vi "Plot Editor.vi"(6 "Original Plot Idx":i32=-1, 7 "Original Graph Name":string, 8 "Error In":errorcluster, 9 "Plot Style in":T2={"Plot Index"=0, "Plot.Bar Plot Style"=0, "Plot.DigitalLineStyle"=1, "Plot.TransitionLocation"=2, "Plot.Transition Type"=0, "Plot.Fill To"=-1, "Plot.Fill/Pt. Color"=16777222, "Plot.Label Format"=3, "Plot.Line Style"=0, "Plot.Line Width"=1, "Plot.Plot Color"=16777222, "Plot.Plot Interpolation"=2, "Plot.Plot Name"="", "Plot.Point Style"=0, "Plot.Visible?"=TRUE, "Plot.XScaleIdx"=0, "Plot.YScaleIdx"=0, "Plot.Anti-aliased"=TRUE}, 10 "Plot in":T3, 11 "Original Graph Refnum":T1) -> (0 "Error Out":errorcluster, 1 "Plot Style out":T2, 2 "Plot out":T3)   [LabVIEW 2019, in "Plot Editor.lvlib"]
uses:
  Plot Editor.lvlib
  XY Graph/XY Graph Plot Properties.ctl
  XY Graph/XY Plot Data.ctl
  XY Graph/XY Graph Refnum.ctl
  Plot Editor Q [Element].ctl
  Plot Editor Q [Event] List.ctl
  Plot Editor Internal Variables.ctl
  <vilib>/Utility/error.llb/DialogType.ctl
  <vilib>/Utility/miscctls.llb/LVPoint32TypeDef.ctl
  XY Graph/XY Graph Add-Ons.lvlib
  Notebook/Notebook.lvlib
  Arrays/Define Ramp Array Dialog.vi
  Rich Text Box/Rich Text Box.lvlib
  Variant/Variant to Data/Variant to Data.lvlib
panel:
  out "Y Array Sum":dbl format="%#_5g"
  out "X Array Sum":dbl format="%#_5g"
  in  "X Array":dbl[](array[numeric])
  in  "Copy":bool
  in  "Cancel":bool
  out "Error":errorcluster
  in  "Reset Style":bool
  out "Y Array Size":i32 format="%#_5g"
  in  "Cancel Data Edit":bool
  in  "OK":bool
  out "X Array Size":i32 format="%#_5g"
  in  "Y Array":dbl[](array[numeric]) caption="X Array"
  out "Plot Preview":cluster{"X Array":dbl[], "Y Array":dbl[]}[](graph)
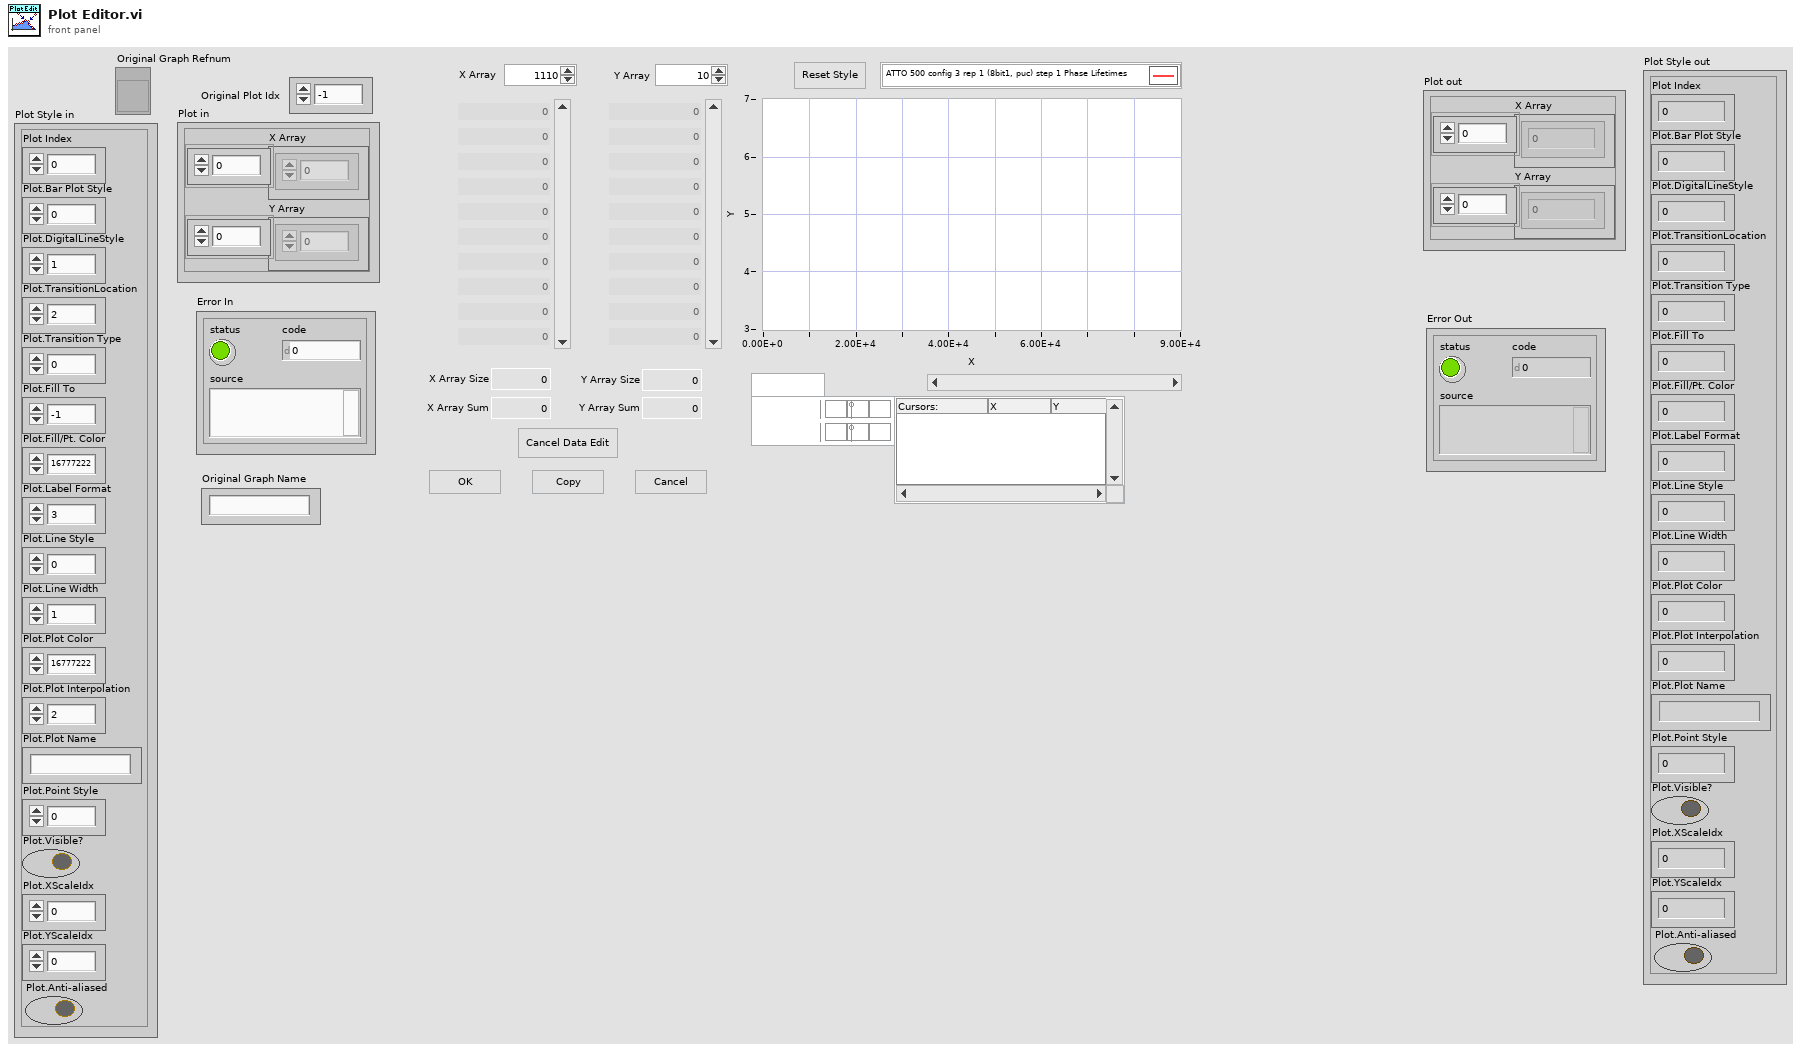
[diagram p1: front panel]
types:
  T1 = typedef "XY Graph Add-Ons.lvlib/XY Graph Refnum.ctl" = refnum<vi>
  T2 = typedef "XY Graph Plot Properties.ctl" = cluster{"Plot Index":i32, "Plot.Bar Plot Style":u8, "Plot.DigitalLineStyle":u8, "Plot.TransitionLocation":u8, "Plot.Transition Type":u8, "Plot.Fill To":i16, "Plot.Fill/Pt. Color":u32, "Plot.Label Format":u8, "Plot.Line Style":u8, "Plot.Line Width":u8, "Plot.Plot Color":u32, "Plot.Plot Interpolation":u8, "Plot.Plot Name":string, "Plot.Point Style":u8, "Plot.Visible?":bool, "Plot.XScaleIdx":u32, "Plot.YScaleIdx":u32, "Plot.Anti-aliased":bool}
  T3 = typedef "XY Plot Data.ctl" = cluster{"X Array":dbl[], "Y Array":dbl[]}
  T4 = typedef "Plot Editor.lvlib/Plot Editor Q [Element].ctl" = cluster{"Plot Editor Q Event":T5, "Data":variant}
  T5 = typedef "Plot Editor.lvlib/Plot Editor Q [Event] List.ctl" = enum16{"Idle", "Initialization", "Controls >> Store", "Store >> Plot", "Update Plot Style", "Check Data Array Alignment", "Reset Data", "Reset Style", "Accept & Quit", "Copy & Quit", "Save Plot", "Load Plot", "Remove out-of-bound Values", "Delete Element", "Insert Element Before", "Insert Element After", "Update output string", "Remove NaN-containing Pairs", "Fill Array with Ramp", "Quit"}
  T6 = typedef "Plot Editor.lvlib/Plot Editor Internal Variables.ctl" = cluster{"X Array":dbl[], "Y Array":dbl[], "XY Plot Properties":T2, "X Array Index Values":u32[], "Y Array Index Values":u32[], "Original XY Plot Properties":T2, "Original X Array":dbl[], "Original Y Array":dbl[], "VI title suffix":string, "Refnum based call":bool}
  T7 = typedef "LVPoint32TypeDef.ctl" = cluster{"Horizontal":i32, "Vertical":i32}
  T8 = typedef "Rich Text Box.lvlib/Text Formatting.ctl" = cluster{"Font":string, "Text Color":T9, "Text Background Color":T9, "Text Style":enum16{"Regular", "Bold", "Italic", "Underline", "Strikeout"}, "Font Size (Points)":dbl, "Text Alignment":i32}
  T9 = typedef "Rich Text Box.lvlib/Text Colors.ctl" = enum16{"Unchanged", "Black", "Blue", "Brown", "Gray", "Green", "Orange", "Pink", "Red", "White"}
  T10 = typedef "DialogType.ctl" = u16
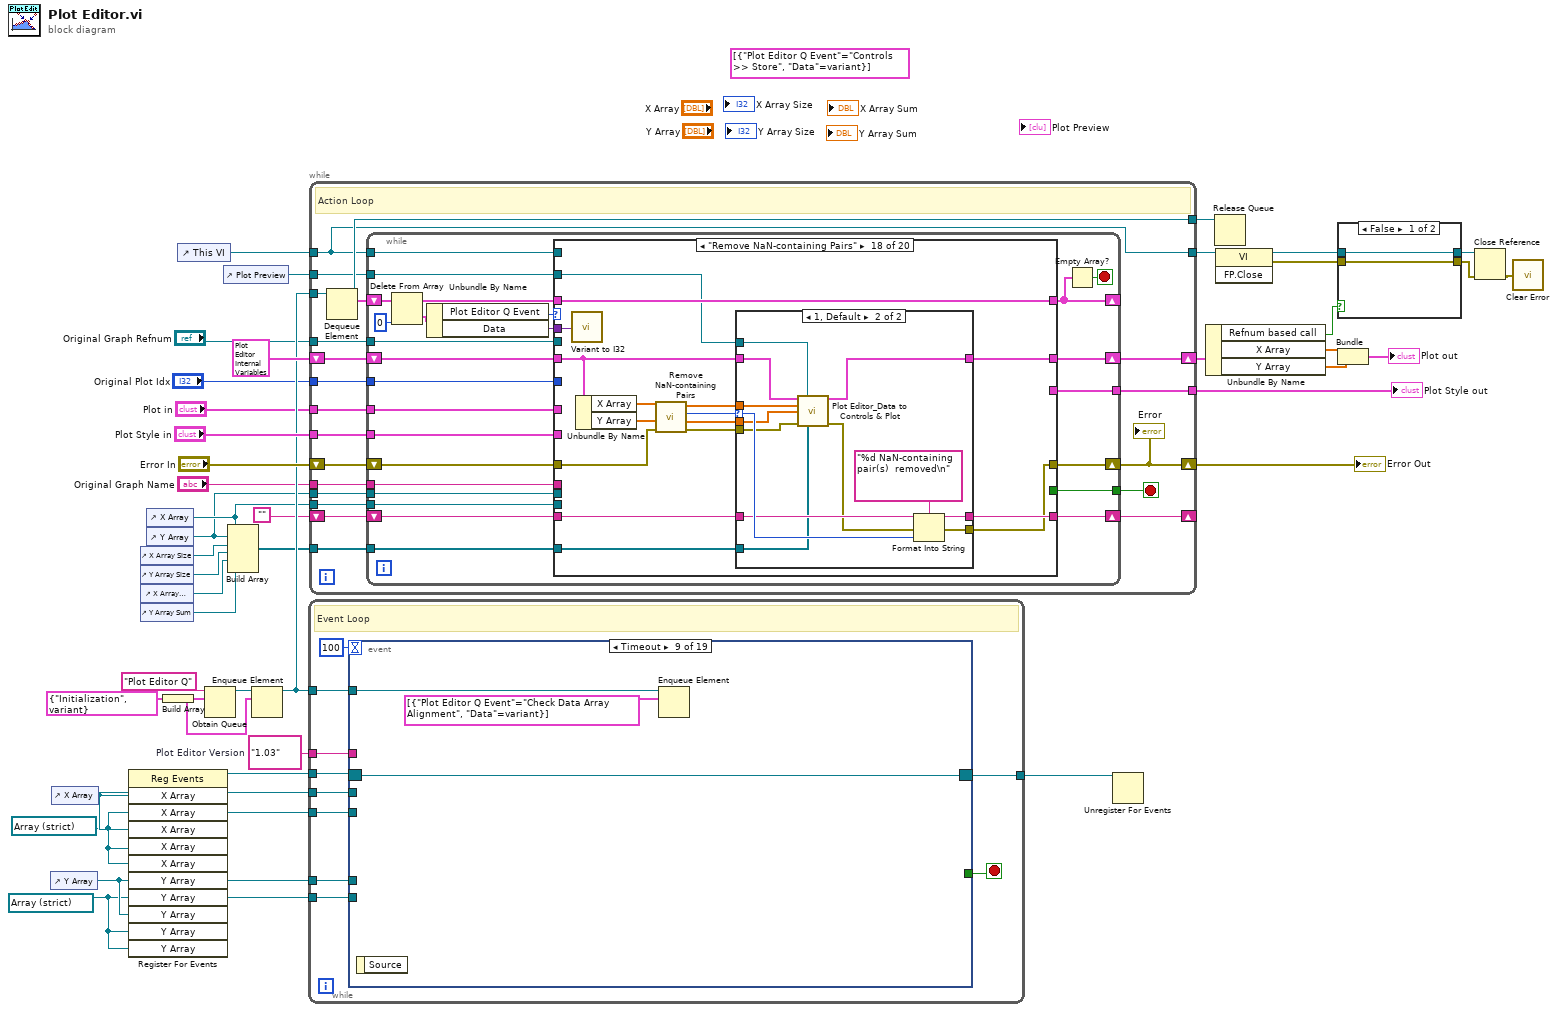
[diagram p0: block diagram]
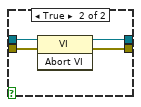
[diagram p2: hidden frame]
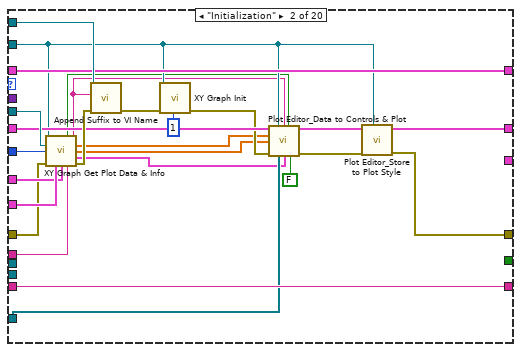
[diagram p4: hidden frame]
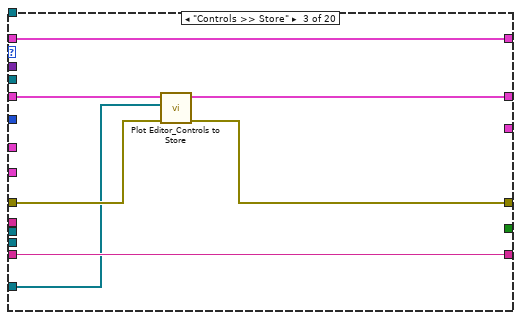
[diagram p5: hidden frame]
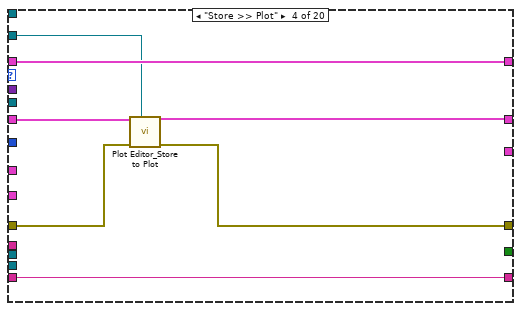
[diagram p6: hidden frame]
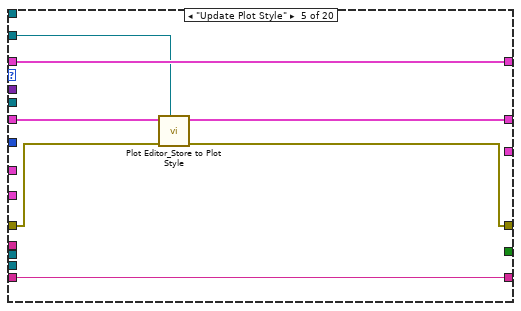
[diagram p7: hidden frame]
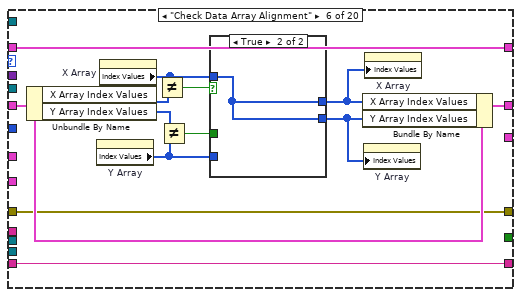
[diagram p8: hidden frame]
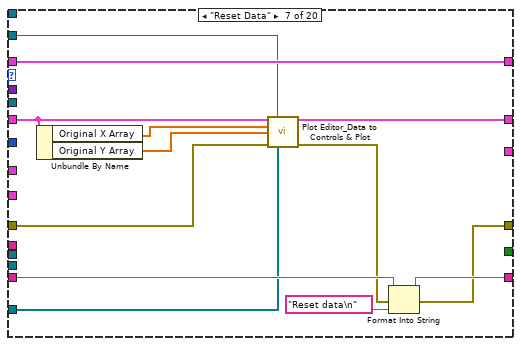
[diagram p11: hidden frame]
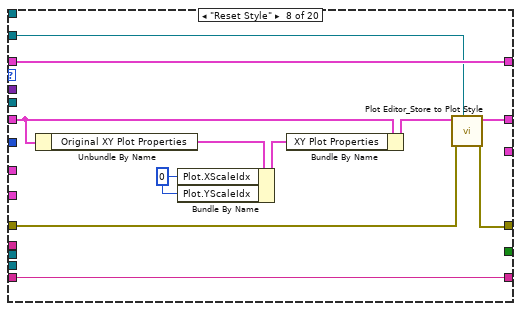
[diagram p12: hidden frame]
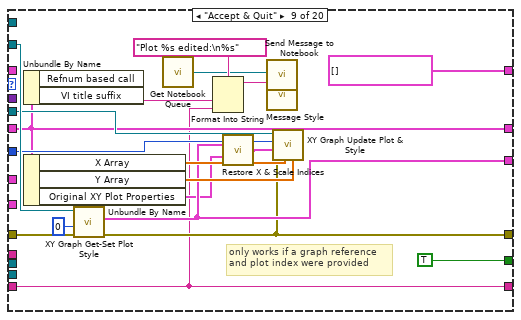
[diagram p13: hidden frame]
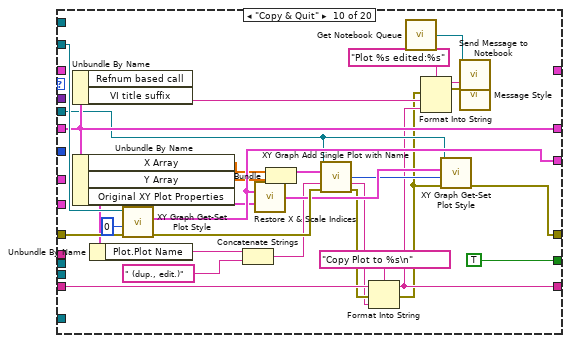
[diagram p14: hidden frame]
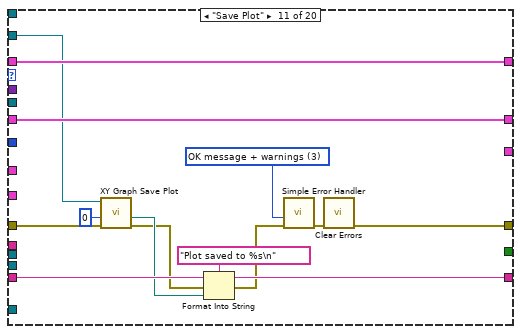
[diagram p15: hidden frame]
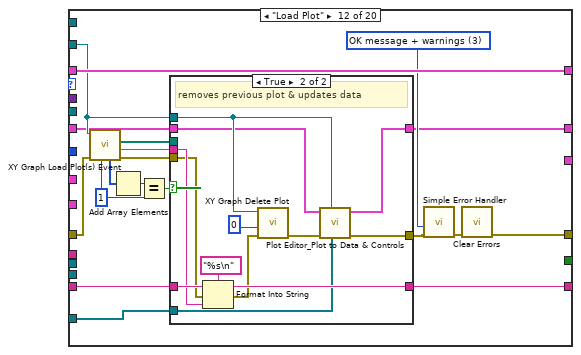
[diagram p16: hidden frame]
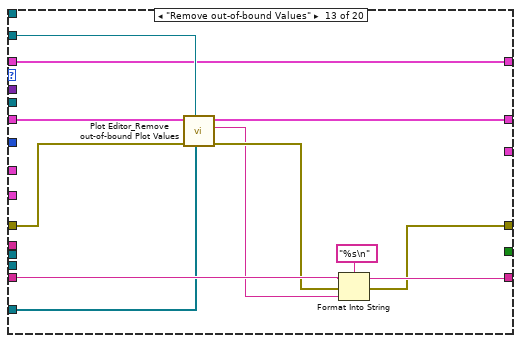
[diagram p18: hidden frame]
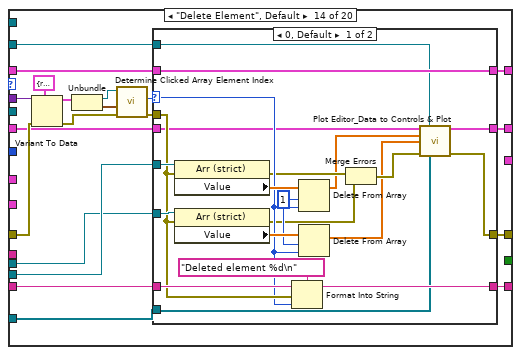
[diagram p19: hidden frame]
diagram:
  w4 = refnum<vi> refnum ("Y Array")
  w3 = refnum<vi> refnum ("X Array")
  (unwired) T4[] [{"Plot Editor Q Event"=enum."Controls >> Store", "Data"=variant}] ("array")
  w27 = "1.03"  # Plot Editor Version
  n1 = control-ref of="Y Array"() -> (w5:refnum<vi>)
  n2 = control-ref of="X Array"() -> (w6:refnum<vi>)
  n3 = register-events(w6, w3, w6, w3, w3, w5, w4, w5, w4, w4) -> (reference out=w26:refnum<event-registration>)  [unwired: 2 in, 1 out]
  n4 = control-ref of="X Array Size"() -> (w9:refnum<vi>)
  n5 = control-ref of="Y Array Size"() -> (w8:refnum<vi>)
  n6 = control-ref of="X Array Sum"() -> (w2:refnum<vi>)
  n7 = control-ref of="Y Array Sum"() -> (w1:refnum<vi>)
  n8 = control-ref of="X Array"() -> (w11:refnum<vi>)
  n9 = control-ref of="Y Array"() -> (w10:refnum<vi>)
  n10 = Build Array(T4 {"Plot Editor Q Event"=enum."Initialization", "Data"=variant} ("Plot Editor Q Element")) -> (w28:T4[])
  n11 = control-ref of="This VI"() -> (w18:refnum<vi>)
  n12 = Obtain Queue(name (unnamed)="Plot Editor Q", element data type=w28) -> (queue out=w41:refnum<queue>)  [unwired: 3 in, 2 out]
  n13 = control-ref of="Plot Preview"() -> (w36:refnum<vi>)
  n14 = Build Array(w11, w10, w9, w8, w2, w1) -> (w7:refnum<vi>[])
  n15 = Enqueue Element(queue=w41, element=w28) -> (queue out=w29:refnum<queue>)  [unwired: 2 in, 2 out]
  n16 = while {
    tunnel: w29 -> [w52]
    tunnel: w27 -> [w51]
    tunnel: w26 -> [w50]
    tunnel: w6 -> [w49]
    tunnel: w5 -> [w48]
    tunnel: [w47] -> w25
    tunnel: w3 -> [w46]
    tunnel: w4 -> [w45]
    stop <- w53 stop-if-true
    # "Event Loop"
    n17 = event shown="[8] Timeout" {
      selector: w50 -> [_ _ _ _ _ w159 w163 w166 w169 w175 w181 w185 w190 _ _ _ _ _ _]
      dyn-events: [_ _ _ _ _ w158 w162 w166 w169 w174 w180 w184 w189 _ _ _ _ _ _] -> w47
      timeout: 100 -> [_ _ _ _ _ _ _ _ _ _ _ _ _ _ _ _ _ _ _]
      tunnel: [w56 w58 _ _ _ _ _ _ _ _ _ _ _ _ _ _ TRUE ("Discard?") TRUE ("Discard?") TRUE ("Discard?")] -> w53
      tunnel: w52 -> [w55 w59 w93 w124 w148 _ _ w165 w168 w171 w176 _ _ w200 w202 w204 w207 w210 w213]
      tunnel: w51 -> [_ w57 _ _ _ _ _ _ _ _ _ _ _ _ _ _ _ _ _]
      tunnel: w49 -> [_ _ _ _ _ w157 _ _ _ w173 _ w183 w188 _ _ _ _ _ _]
      tunnel: w48 -> [_ _ _ _ _ _ w161 _ _ _ w178 _ w187 _ _ _ _ _ _]
      tunnel: w46 -> [_ _ _ _ _ w156 _ _ _ w172 _ w182 _ _ _ _ _ _ _]
      tunnel: w45 -> [_ _ _ _ _ _ w160 _ _ _ w179 _ w186 _ _ _ _ _ _]
      event Panel Close? {
        w56 = TRUE ("Discard?")
        n18 = event-data() -> ()  [unwired: 1 in, 1 out]
        n19 = Enqueue Element(queue=w55, element=T4[] [{"Plot Editor Q Event"=enum."Quit", "Data"=variant}]) -> ()  [unwired: 2 in, 3 out]
        n20 = event-data("Discard?"=w56) -> ()  [unwired: 1 in, 1 out]
      }
      event Menu Selection (User) {
        n21 = event-data() -> ("ItemTag"=w60:string)  [unwired: 1 in]
        n22 = case shown="\"About...\"" w60 {
          tunnel: w59 -> [_ w62 w64 w68 w81 _]
          tunnel: [_ _ _ w65 _ _] -> w58
          tunnel: w57 -> [_ _ _ _ _ w86]
          frame "", Default {
          }
          frame "Save Plot" {
            n23 = Enqueue Element(queue=w62, element=T4[] [{"Plot Editor Q Event"=enum."Save Plot", "Data"=variant}]) -> ()  [unwired: 2 in, 3 out]
          }
          frame "Load Plot" {
            n24 = Enqueue Element(queue=w64, element=T4[] [{"Plot Editor Q Event"=enum."Load Plot", "Data"=variant}]) -> ()  [unwired: 2 in, 3 out]
          }
          frame "Quit" {
            n25 = call "Two Buttons Dialog Window.vi"("OK Button Text"="Accept & Quit" ("T button name (\"OK\")"), "Message"="Are you sure you want to quit Plot Editor?\nQuitting will save the current changes and return to the original graph." ("message")) -> ("OK?"=w65:bool)  [unwired: 1 in]
            n26 = case shown="True" w65 {
              tunnel: w68 -> [_ w70]
              frame False {
              }
              frame True {
                n27 = Enqueue Element(queue=w70, element=T4[] [{"Plot Editor Q Event"=enum."Accept & Quit", "Data"=variant}]) -> ()  [unwired: 2 in, 3 out]
              }
            }
          }
          frame "Paste Data from Clipboard" {
            w72 = "\n"
            n28 = invoke class="App" method="Clipboard.Read"() -> ("Read Clipbrd"=w78:string)  [unwired: 3 in, 2 out]
            n29 = call <userlib>:"String to 1D Array__ogtk.vi"("delimiter (Tab)"=w72, "string"=w78) -> ("Array of Strings"=w77:string[])  [unwired: 9 in]
            n30 = Delete From Array(array=w77, length=1, index=0) -> (array with subset deleted=w74:string[])  [unwired: 1 out]
            n31 = call <userlib>:"1D Array to String__ogtk.vi"("delimiter (Tab)"=w72, "Array of Strings"=w74) -> ("delimited string"=w73:string)  [unwired: 9 in]
            n32 = Spreadsheet String To Array(format string="%#g", spreadsheet string=w73) -> (array=w84:dbl[][])  [unwired: 2 in]
            n33 = Transpose 2D Array(2D array=w84) -> (transposed array=w71:dbl[][])
            n34 = Enqueue Element(queue=w81, element=T4[] [{"Plot Editor Q Event"=enum."Controls >> Store", "Data"=variant}, {"Plot Editor Q Event"=enum."Store >> Plot", "Data"=variant}]) -> ()  [unwired: 2 in, 3 out]
            n35 = Index Array(array=w71) -> (element #1=w83:dbl[], element #2=w82:dbl[])  [unwired: 4 in]
            n36 = local write "X Array"(w83) -> ()
            n37 = local write "Y Array"(w82) -> ()
          }
          frame "About..." {
            n38 = Format Into String(format string="                                      Plot Editor\n                                      version %s\n\n                              Author: X. Michalet\n(c) 2017-2020 The Regents of the  University of California" ("message"), w86) -> (resulting string=w85:string)  [unwired: 2 in, 1 out]
            n39 = One Button Dialog(message=w85) -> ()  [unwired: 1 in, 1 out]
          }
        }
      }
      event "X Array": Shortcut Menu Selection (User) {
        n40 = event-data() -> ("ItemTag"=w94:string, "CtlRef"=w91:refnum<vi>, "Coords"=w90:T7)  [unwired: 1 in]
        n41 = case shown="\"Remove NaN-containing Pairs\"" w94 {
          tunnel: [w95 w101 w107 w113 w116 w118] -> w92
          tunnel: w91 -> [_ w100 w106 w112 _ _]
          tunnel: w90 -> [_ w99 w105 w111 _ _]
          frame "", Default {
            n42 = Build Array(T4 {"Plot Editor Q Event"=enum."Idle", "Data"=variant} ("Plot Editor Q Element")) -> (w95:T4[])
          }
          frame "Delete Element" {
            n43 = Bundle("CtlRef"=w100, "Coords"=w99) -> (w97:cluster{"CtlRef":refnum<vi>, "Coords":T7})  [unwired: 1 in]
            n44 = Bundle By Name(cluster=T4 {"Plot Editor Q Event"=enum."Delete Element", "Data"=variant} ("Plot Editor Q Element"), "Data"=w97) -> (w98:T4)
            n45 = Build Array(w98) -> (w101:T4[])
          }
          frame "Insert Element Before" {
            n46 = Bundle("CtlRef"=w106, "Coords"=w105) -> (w103:cluster{"CtlRef":refnum<vi>, "Coords":T7})  [unwired: 1 in]
            n47 = Bundle By Name(cluster=T4 {"Plot Editor Q Event"=enum."Insert Element Before", "Data"=variant} ("Plot Editor Q Element"), "Data"=w103) -> (w104:T4)
            n48 = Build Array(w104) -> (w107:T4[])
          }
          frame "Insert Element After" {
            n49 = Bundle("CtlRef"=w112, "Coords"=w111) -> (w109:cluster{"CtlRef":refnum<vi>, "Coords":T7})  [unwired: 1 in]
            n50 = Bundle By Name(cluster=T4 {"Plot Editor Q Event"=enum."Insert Element After", "Data"=variant} ("Plot Editor Q Element"), "Data"=w109) -> (w110:T4)
            n51 = Build Array(w110) -> (w113:T4[])
          }
          frame "Fill Array with Ramp" {
            n52 = Build Array(T4 {"Plot Editor Q Event"=enum."Fill Array with Ramp", "Data"=variant} ("Plot Editor Q Element")) -> (w116:T4[])
          }
          frame "Remove NaN-containing Pairs" {
            n53 = Build Array(T4 {"Plot Editor Q Event"=enum."Remove NaN-containing Pairs", "Data"=variant} ("Plot Editor Q Element")) -> (w118:T4[])
          }
        }
        n54 = Build Array (concatenate)(w92, T4[] [{"Plot Editor Q Event"=enum."Controls >> Store", "Data"=variant}, {"Plot Editor Q Event"=enum."Store >> Plot", "Data"=variant}] ("array")) -> (w89:T4[])
        n55 = Enqueue Element(queue=w93, element=w89) -> ()  [unwired: 2 in, 3 out]
      }
      event "Y Array": Shortcut Menu Selection (User) {
        n56 = event-data() -> ("ItemTag"=w125:string, "CtlRef"=w123:refnum<vi>, "Coords"=w122:T7)  [unwired: 1 in]
        n57 = case shown="\"Remove NaN-containing Pairs\"" w125 {
          tunnel: [w126 w130 w136 w142 w147] -> w121
          tunnel: w123 -> [_ w129 w135 w141 _]
          tunnel: w122 -> [_ w128 w134 w140 _]
          frame "", Default {
            n58 = Build Array(T4 {"Plot Editor Q Event"=enum."Idle", "Data"=variant} ("Plot Editor Q Element")) -> (w126:T4[])
          }
          frame "Delete Element" {
            n59 = Bundle("CtlRef"=w129, "Coords"=w128) -> (w132:cluster{"CtlRef":refnum<vi>, "Coords":T7})  [unwired: 1 in]
            n60 = Bundle By Name(cluster=T4 {"Plot Editor Q Event"=enum."Delete Element", "Data"=variant} ("Plot Editor Q Element"), "Data"=w132) -> (w133:T4)
            n61 = Build Array(w133) -> (w130:T4[])
          }
          frame "Insert Element Before" {
            n62 = Bundle("CtlRef"=w135, "Coords"=w134) -> (w138:cluster{"CtlRef":refnum<vi>, "Coords":T7})  [unwired: 1 in]
            n63 = Bundle By Name(cluster=T4 {"Plot Editor Q Event"=enum."Insert Element Before", "Data"=variant} ("Plot Editor Q Element"), "Data"=w138) -> (w139:T4)
            n64 = Build Array(w139) -> (w136:T4[])
          }
          frame "Insert Element After" {
            n65 = Bundle("CtlRef"=w141, "Coords"=w140) -> (w144:cluster{"CtlRef":refnum<vi>, "Coords":T7})  [unwired: 1 in]
            n66 = Bundle By Name(cluster=T4 {"Plot Editor Q Event"=enum."Insert Element After", "Data"=variant} ("Plot Editor Q Element"), "Data"=w144) -> (w145:T4)
            n67 = Build Array(w145) -> (w142:T4[])
          }
          frame "Remove NaN-containing Pairs" {
            n68 = Build Array(T4 {"Plot Editor Q Event"=enum."Remove NaN-containing Pairs", "Data"=variant} ("Plot Editor Q Element")) -> (w147:T4[])
          }
        }
        n69 = Build Array (concatenate)(w121, T4[] [{"Plot Editor Q Event"=enum."Controls >> Store", "Data"=variant}, {"Plot Editor Q Event"=enum."Store >> Plot", "Data"=variant}] ("array")) -> (w120:T4[])
        n70 = Enqueue Element(queue=w124, element=w120) -> ()  [unwired: 2 in, 3 out]
      }
      event "Plot Preview": Shortcut Menu Selection (User) {
        n71 = event-data() -> ("ItemTag"=w149:string)  [unwired: 1 in, 1 out]
        n72 = case shown="\"Remove out-of-bound Values\"" w149 {
          tunnel: w148 -> [_ w151 w153 w155]
          frame "", Default {
          }
          frame "Save Plot" {
            n73 = Enqueue Element(queue=w151, element=T4[] [{"Plot Editor Q Event"=enum."Save Plot", "Data"=variant}]) -> ()  [unwired: 2 in, 3 out]
          }
          frame "Load Plot" {
            n74 = Enqueue Element(queue=w153, element=T4[] [{"Plot Editor Q Event"=enum."Load Plot", "Data"=variant}]) -> ()  [unwired: 2 in, 3 out]
          }
          frame "Remove out-of-bound Values" {
            n75 = Enqueue Element(queue=w155, element=T4[] [{"Plot Editor Q Event"=enum."Remove out-of-bound Values", "Data"=variant}]) -> ()  [unwired: 2 in, 3 out]
          }
        }
      }
      event Mouse Down {
        n76 = event-data() -> ()  [unwired: 1 in, 1 out]
        n77 = register-events(reference=w159, w156, w157, w157, w157) -> (reference out=w158:refnum<event-registration>)  [unwired: 7 in, 1 out]
      }
      event Mouse Down {
        n78 = event-data() -> ()  [unwired: 1 in, 1 out]
        n79 = register-events(reference=w163, w160, w161, w161, w161) -> (reference out=w162:refnum<event-registration>)  [unwired: 7 in, 1 out]
      }
      event Mouse Move; Mouse Wheel {
        n80 = event-data() -> ()  [unwired: 1 in, 1 out]
        n81 = Enqueue Element(queue=w165, element=T4[] [{"Plot Editor Q Event"=enum."Check Data Array Alignment", "Data"=variant}]) -> ()  [unwired: 2 in, 3 out]
      }
      event Timeout {
        n82 = event-data() -> ()  [unwired: 1 in, 1 out]
        n83 = Enqueue Element(queue=w168, element=T4[] [{"Plot Editor Q Event"=enum."Check Data Array Alignment", "Data"=variant}]) -> ()  [unwired: 2 in, 3 out]
      }
      event Mouse Up {
        n84 = event-data() -> ()  [unwired: 1 in, 1 out]
        n85 = register-events(reference=w175, w173, w172, w172) -> (reference out=w174:refnum<event-registration>)  [unwired: 8 in, 1 out]
        n86 = Enqueue Element(queue=w171, element=T4[] [{"Plot Editor Q Event"=enum."Check Data Array Alignment", "Data"=variant}]) -> ()  [unwired: 2 in, 3 out]
      }
      event Mouse Up {
        n87 = event-data() -> ()  [unwired: 1 in, 1 out]
        n88 = register-events(reference=w181, w178, w179, w179) -> (reference out=w180:refnum<event-registration>)  [unwired: 8 in, 1 out]
        n89 = Enqueue Element(queue=w176, element=T4[] [{"Plot Editor Q Event"=enum."Check Data Array Alignment", "Data"=variant}]) -> ()  [unwired: 2 in, 3 out]
      }
      event Mouse Leave {
        n90 = event-data() -> ()  [unwired: 1 in, 1 out]
        n91 = register-events(reference=w185, w183, w182, w182, w182) -> (reference out=w184:refnum<event-registration>)  [unwired: 7 in, 1 out]
      }
      event Mouse Leave {
        n92 = event-data() -> ()  [unwired: 1 in, 1 out]
        n93 = register-events(reference=w190, w188, w187, w186, w186, w186) -> (reference out=w189:refnum<event-registration>)  [unwired: 6 in, 1 out]
      }
      event "X Array", "Y Array": Value Change {
        n94 = event-data() -> ("CtlRef"=w195:refnum<vi>)  [unwired: 1 in]
        n95 = property class="Arr (strict)"(reference=w195) -> (error out=w192:errorcluster, "Label.Text"=w193:string)  [unwired: 1 in, 1 out]
        n96 = Format Into String(format string="User added %s data", error in=w192, w193) -> (resulting string=w191:string)  [unwired: 1 in, 1 out]
        n97 = Bundle By Name(cluster=T4 {"Plot Editor Q Event"=enum."Update output string", "Data"=variant} ("Plot Editor Q Element"), "Data"=w191) -> (w196:T4)
        n98 = Build Array (concatenate)(T4[] [{"Plot Editor Q Event"=enum."Controls >> Store", "Data"=variant}, {"Plot Editor Q Event"=enum."Store >> Plot", "Data"=variant}, {"Plot Editor Q Event"=enum."Check Data Array Alignment", "Data"=variant}] ("element"), w196) -> (w198:T4[])
        n99 = Enqueue Element(queue=w200, element=w198) -> ()  [unwired: 2 in, 3 out]
      }
      event "Reset Style": Value Change {
        n100 = event-data() -> ()  [unwired: 1 in, 1 out]
        n101 = Enqueue Element(queue=w202, element=T4[] [{"Plot Editor Q Event"=enum."Reset Style", "Data"=variant}]) -> ()  [unwired: 2 in, 3 out]
      }
      event "Cancel Data Edit": Value Change {
        n102 = event-data() -> ()  [unwired: 1 in, 1 out]
        n103 = Enqueue Element(queue=w204, element=T4[] [{"Plot Editor Q Event"=enum."Reset Data", "Data"=variant}]) -> ()  [unwired: 2 in, 3 out]
      }
      event "OK": Value Change {
        n104 = event-data() -> ()  [unwired: 1 in, 1 out]
        n105 = Enqueue Element(queue=w207, element=T4[] [{"Plot Editor Q Event"=enum."Accept & Quit", "Data"=variant}]) -> ()  [unwired: 2 in, 3 out]
      }
      event "Copy": Value Change {
        n106 = event-data() -> ()  [unwired: 1 in, 1 out]
        n107 = Enqueue Element(queue=w210, element=T4[] [{"Plot Editor Q Event"=enum."Copy & Quit", "Data"=variant}]) -> ()  [unwired: 2 in, 3 out]
      }
      event "Cancel": Value Change {
        n108 = event-data() -> ()  [unwired: 1 in, 1 out]
        n109 = Enqueue Element(queue=w213, element=T4[] [{"Plot Editor Q Event"=enum."Quit", "Data"=variant}]) -> ()  [unwired: 2 in, 3 out]
      }
    }
  }
  n110 = while {
    tunnel: w29 -> [w234]
    tunnel: [w231] -> w40
    shift-right: [w228] -> w34
    shift-left: T6 {"X Array"=[], "Y Array"=[], "XY Plot Properties"={"Plot Index"=0, "Plot.Bar Plot Style"=0, "Plot.DigitalLineStyle"=0, "Plot.TransitionLocation"=0, "Plot.Transition Type"=0, "Plot.Fill To"=-1, "Plot.Fill/Pt. Color"=0, "Plot.Label Format"=0, "Plot.Line Style"=0, "Plot.Line Width"=0, "Plot.Plot Color"=0, "Plot.Plot Interpolation"=0, "Plot.Plot Name"="Plot", "Plot.Point Style"=0, "Plot.Visible?"=FALSE, "Plot.XScaleIdx"=0, "Plot.YScaleIdx"=0, "Plot.Anti-aliased"=FALSE}, "X Array Index Values"=[], "Y Array Index Values"=[], "Original XY Plot Properties"={"Plot Index"=0, "Plot.Bar Plot Style"=0, "Plot.DigitalLineStyle"=0, "Plot.TransitionLocation"=0, "Plot.Transition Type"=0, "Plot.Fill To"=0, "Plot.Fill/Pt. Color"=0, "Plot.Label Format"=0, "Plot.Line Style"=0, "Plot.Line Width"=0, "Plot.Plot Color"=0, "Plot.Plot Interpolation"=0, "Plot.Plot Name"="", "Plot.Point Style"=0, "Plot.Visible?"=FALSE, "Plot.XScaleIdx"=0, "Plot.YScaleIdx"=0, "Plot.Anti-aliased"=FALSE}, "Original X Array"=[], "Original Y Array"=[], "VI title suffix"="", "Refnum based call"=FALSE} ("Plot Editor Internal Data") -> [w230]
    shift-right: [w219] -> w35
    shift-left: "Error In" -> [w227]
    tunnel: "Plot Style in" -> [w229]
    tunnel: w36 -> [w226]
    tunnel: [w225] -> w30
    tunnel: "Original Graph Refnum" -> [w224]
    tunnel: "Original Plot Idx" -> [w223]
    tunnel: "Plot in" -> [w222]
    tunnel: "Original Graph Name" -> [w221]
    tunnel: w18 -> [w220]
    tunnel: [w220] -> w20
    shift-right: [w217] -> _
    shift-left: "" -> [w218]
    tunnel: w11 -> [w216]
    tunnel: w10 -> [w215]
    tunnel: w7 -> [w214]
    stop <- w232 stop-if-true
    # "Action Loop"
    n111 = Dequeue Element(queue=w234) -> (queue out=w231:refnum<queue>, element=w233:T4[])  [unwired: 2 in, 2 out]
    n112 = while {
      tunnel: [w260] -> w232
      shift-right: [w256] -> _
      shift-left: w233 -> [w259]
      tunnel: w229 -> [w253]
      tunnel: w226 -> [w235]
      shift-right: [w252] -> w228
      shift-left: w230 -> [w254]
      shift-right: [w248] -> w219
      shift-left: w227 -> [w249]
      tunnel: [w247] -> w225
      tunnel: w224 -> [w246]
      tunnel: w223 -> [w245]
      tunnel: w222 -> [w244]
      tunnel: w221 -> [w243]
      tunnel: w220 -> [w242]
      shift-right: [w239] -> w217
      shift-left: w218 -> [w240]
      tunnel: w216 -> [w238]
      tunnel: w215 -> [w237]
      tunnel: w214 -> [w236]
      stop <- w255 stop-if-true
      n113 = Delete From Array(array=w259, index=0) -> (deleted portion=w251:T4, array with subset deleted=w257:T4[])  [unwired: 1 in]
      n114 = Unbundle By Name(w251) -> ("Plot Editor Q Event"=w250:T5, "Data"=w241:variant)
      n115 = case shown="\"Remove NaN-containing Pairs\"" w250 {
        tunnel: [_ _ _ _ _ _ _ _ TRUE TRUE _ _ _ _ _ _ _ _ _ TRUE] -> w260
        tunnel: w257 -> [w264 w279 w297 w304 w311 w318 w343 w357 _ _ w421 w440 w460 w476 w521 w566 w613 w618 w651 _]
        tunnel: [w264 w279 w297 w304 w311 w318 w343 w357 T4[] [] _ w421 w440 w460 w475 w520 w565 w613 w618 w648 T4[] []] -> w256
        tunnel: w254 -> [w262 w276 w295 w300 w307 w320 w340 w356 w370 w405 w420 w429 w459 w472 w517 w562 w605 w617 w658 w687]
        tunnel: w253 -> [_ w288 _ _ _ _ _ _ _ _ _ _ _ _ _ _ _ _ _ _]
        tunnel: [w262 w277 w294 w301 w306 w319 w339 w350 w370 w405 w420 w428 w458 w469 w516 w561 w605 w615 w657 w688] -> w252
        tunnel: w249 -> [w263 w286 w292 w298 w310 w315 w338 w349 w368 w403 w418 w439 w468 w473 w519 w564 w607 w623 w656 _]
        tunnel: [w263 w278 w293 w299 w309 w315 w342 w348 w366 w399 w415 w436 w463 w474 w518 w563 w608 w621 w649 _] -> w248
        tunnel: [_ _ _ _ _ _ _ _ w367 w402 _ _ _ _ _ _ _ _ _ w684] -> w247
        tunnel: w246 -> [_ w290 _ _ _ _ _ _ w374 w398 _ _ _ _ _ _ _ _ _ _]
        tunnel: w245 -> [_ w289 _ _ _ _ _ _ w373 _ _ _ _ _ _ _ _ _ _ _]
        tunnel: w244 -> [_ w287 _ _ _ _ _ _ _ _ _ _ _ _ _ _ _ _ _ _]
        tunnel: w243 -> [_ w285 _ _ _ _ _ _ _ _ _ _ _ _ _ _ _ _ _ _]
        tunnel: w242 -> [_ w284 _ _ _ _ _ _ _ _ _ _ _ _ _ _ _ _ _ _]
        tunnel: w241 -> [_ _ _ _ _ _ _ _ _ _ _ _ _ w488 w533 w578 w612 w629 _ _]
        tunnel: w238 -> [_ _ _ _ _ _ _ _ _ _ _ _ _ w482 w527 w575 _ _ _ _]
        tunnel: w237 -> [_ _ _ _ _ _ _ _ _ _ _ _ _ w481 w526 w574 _ _ _ _]
        tunnel: w240 -> [w261 w281 w296 w303 w308 w314 w346 w352 w358 w388 w413 w426 w467 w478 w523 w568 w611 w625 w653 w682]
        tunnel: [w261 w281 w296 w303 w308 w314 w345 w352 w358 w381 w410 w425 w466 w477 w522 w567 w610 w624 w652 w682] -> w239
        tunnel: w236 -> [_ w271 w291 _ _ _ w334 _ _ _ _ w422 w457 w471 w514 w560 _ w616 w647 _]
        tunnel: w235 -> [_ w274 _ w302 w305 _ w335 w347 w376 w407 w419 w431 w462 w470 w515 w559 _ w614 w646 _]
        frame "Idle" {
        }
        frame "Initialization" {
          n116 = call "XY Graph Get Plot Data & Info.vi"("Destination Graph"=w274, "Original Graph"=w290, "Original Plot Idx"=w289, "Error In"=w286, "Plot Style in"=w288, "Plot in"=w287, "Graph Origin Name"=w285) -> ("Refnum based call"=w265:bool, "VI Title Suffix"=w266:string, "X Array"=w270:dbl[], "Y Array"=w269:dbl[], "Plot Style out"=w267:T2, "Error Out"=w283:errorcluster)  [unwired: 3 in]
          n117 = call "Append Suffix to VI Name.vi"("error in (no error)"=w283, "VI Title Suffix"=w266, "VI in"=w284) -> ("Error Out"=w280:errorcluster)  [unwired: 8 in]
          n118 = call "XY Graph Init.vi"("Max Legend Size (8)"=1 ("Plot.XScaleIdx"), "Error In"=w280, "XYGraph in"=w274) -> ("Error Out"=w273:errorcluster)  [unwired: 8 in]
          n119 = call "Plot Editor_Data to Controls & Plot.vi"("Plot Editor Internal Data"=w276, "XYGraph in"=w274, "VI Title Suffix"=w266, "Refnum based call"=w265, "X Array"=w270, "Y Array"=w269, "error in (no error)"=w273, "Control Refnums"=w271, "Plot Style"=w267, "Data only (T)"=FALSE) -> ("Plot Editor Internal Data"=w275:T6, "error out"=w272:errorcluster)  [unwired: 4 in]
          n120 = call "Plot Editor_Store to Plot Style.vi"("XYGraph in"=w274, "error in (no error)"=w272, "Plot Editor Internal Data"=w275) -> ("error out"=w278:errorcluster, "Plot Editor Internal Data (dup)"=w277:T6)  [unwired: 7 in]
        }
        frame "Controls >> Store" {
          n121 = call "Plot Editor_Controls to Store.vi"("Error In"=w292, "Control Refnums"=w291, "Plot Editor Internal Data in"=w295) -> ("Error Out"=w293:errorcluster, "Plot Editor Internal Data out"=w294:T6)  [unwired: 7 in]
        }
        frame "Store >> Plot" {
          n122 = call "Plot Editor_Store to Plot.vi"("XYGraph in"=w302, "Error In"=w298, "Plot Editor Internal Data"=w300) -> ("Error Out"=w299:errorcluster, "Plot Editor Internal Data (dup)"=w301:T6)  [unwired: 7 in]
        }
        frame "Update Plot Style" {
          n123 = call "Plot Editor_Store to Plot Style.vi"("XYGraph in"=w305, "error in (no error)"=w310, "Plot Editor Internal Data"=w307) -> ("error out"=w309:errorcluster, "Plot Editor Internal Data (dup)"=w306:T6)  [unwired: 7 in]
        }
        frame "Check Data Array Alignment" {
          n124 = Unbundle By Name(w320) -> ("X Array Index Values"=w324:u32[], "Y Array Index Values"=w323:u32[])
          n125 = property on="Y Array" class="Arr (strict)"() -> ("Index Values"=w316:u32[])  [unwired: 2 in, 2 out]
          n126 = property on="X Array" class="Arr (strict)"() -> ("Index Values"=w321:u32[])  [unwired: 2 in, 2 out]
          n127 = Not Equal?(x=w321, y=w324) -> (x != y?=w322:bool)
          n128 = Not Equal?(x=w323, y=w316) -> (x != y?=w317:bool)
          n129 = case shown="True" w322 {
            tunnel: w321 -> [w325 w333]
            tunnel: [w326 w333] -> w312
            tunnel: [w327 w333] -> w313
            tunnel: w317 -> [w329 _]
            tunnel: w316 -> [w328 _]
            frame False {
              n130 = case shown="False" w329 {
                tunnel: w328 -> [w330 w332]
                tunnel: [w331 w332] -> w327
                tunnel: [w330 w332] -> w326
                tunnel: w325 -> [w331 _]
                frame False {
                }
                frame True {
                }
              }
            }
            frame True {
            }
          }
          n131 = Bundle By Name(cluster=w320, "X Array Index Values"=w313, "Y Array Index Values"=w312) -> (w319:T6)
          n132 = property on="Y Array" class="Arr (strict)"("Index Values"=w312) -> ()  [unwired: 2 in, 2 out]
          n133 = property on="X Array" class="Arr (strict)"("Index Values"=w313) -> ()  [unwired: 2 in, 2 out]
        }
        frame "Reset Data" {
          n134 = Unbundle By Name(w340) -> ("Original X Array"=w341:dbl[], "Original Y Array"=w337:dbl[])
          n135 = call "Plot Editor_Data to Controls & Plot.vi"("Plot Editor Internal Data"=w340, "XYGraph in"=w335, "X Array"=w341, "Y Array"=w337, "error in (no error)"=w338, "Control Refnums"=w334) -> ("Plot Editor Internal Data"=w339:T6, "error out"=w336:errorcluster)  [unwired: 8 in]
          n136 = Format Into String(initial string=w346, error in=w336, "Reset data\n" ("format string")) -> (resulting string=w345:string, error out=w342:errorcluster)  [unwired: 1 in]
        }
        frame "Reset Style" {
          w353 = u32 0 ("Plot.XScaleIdx")
          n137 = Unbundle By Name(w356) -> ("Original XY Plot Properties"=w355:T2)
          n138 = Bundle By Name(cluster=w355, "Plot.XScaleIdx"=w353, "Plot.YScaleIdx"=w353) -> (w354:T2)
          n139 = Bundle By Name(cluster=w356, "XY Plot Properties"=w354) -> (w351:T6)
          n140 = call "Plot Editor_Store to Plot Style.vi"("XYGraph in"=w347, "error in (no error)"=w349, "Plot Editor Internal Data"=w351) -> ("error out"=w348:errorcluster, "Plot Editor Internal Data (dup)"=w350:T6)  [unwired: 7 in]
        }
        frame "Accept & Quit" {
          # "only works if a graph reference\nand plot index were provided"
          n141 = Unbundle By Name(w370) -> ("VI title suffix"=w369:string)  [unwired: 1 out]
          n142 = Unbundle By Name(w370) -> ("X Array"=w372:dbl[], "Y Array"=w371:dbl[], "Original XY Plot Properties"=w363:T2)
          n143 = call "XY Graph Get-Set Plot Style.vi"("Error In"=w368, "Plot Index"=0, "XYGraph in"=w376) -> ("Error Out"=w366:errorcluster, "Plot Style out"=w367:T2)  [unwired: 5 in, 2 out]
          n144 = call "Get Notebook Queue.vi"() -> ("Notebook Queue"=w359:refnum<queue>)  [unwired: 9 in]
          n145 = Format Into String(format string="Plot %s edited:\n%s", w369, w358) -> (resulting string=w360:string)  [unwired: 2 in, 1 out]
          n146 = call "Restore X & Scale Indices.vi"("New Plot Style in"=w367, "Original Plot Style in"=w363) -> ("Updated Plot Style out"=w364:T2)  [unwired: 13 in]
          n147 = call "Message Style.vi"() -> ("Message Formatting"=w361:T8)
          n148 = call "Send Message to Notebook.vi"("Notebook Queue"=w359, "Message"=w360, "Text Formatting"=w361) -> ()  [unwired: 16 in, 1 out]
          n149 = call "XY Graph Update Plot & Style.vi"("Y Array"=w371, "X Array"=w372, "Error In"=w366, "XY Plot Style in"=w364, "Plot Idx"=w373, "XY Graph refnum"=w374) -> ()  [unwired: 3 in, 3 out]
        }
        frame "Copy & Quit" {
          n150 = Unbundle By Name(w405) -> ("VI title suffix"=w404:string)  [unwired: 1 out]
          n151 = Unbundle By Name(w405) -> ("X Array"=w393:dbl[], "Y Array"=w392:dbl[], "Original XY Plot Properties"=w390:T2)
          n152 = Unbundle By Name(w390) -> ("Plot.Plot Name"=w389:string)
          n153 = call "XY Graph Get-Set Plot Style.vi"("Error In"=w403, "Plot Index"=0, "XYGraph in"=w407) -> ("Error Out"=w400:errorcluster, "Plot Style out"=w402:T2)  [unwired: 5 in, 2 out]
          n154 = Concatenate Strings(w389, " (dup., edit.)" ("string")) -> (w394:string)
          n155 = call "Restore X & Scale Indices.vi"("New Plot Style in"=w402, "Original Plot Style in"=w390) -> ("Updated Plot Style out"=w397:T2)  [unwired: 13 in]
          n156 = Bundle("X Array"=w393, "Y Array"=w392) -> (w391:cluster{"X Array":dbl[], "Y Array":dbl[]})  [unwired: 1 in]
          n157 = call "XY Graph Add Single Plot with Name.vi"("XYGraph Ref in"=w398, "Plot"=w391, "Plot Name (\"Plot\")"=w394, "error in (no error)"=w400) -> ("Plot Index"=w396:i32, "Plot Name"=w382:string, "error out"=w384:errorcluster)  [unwired: 8 in, 1 out]
          n158 = Format Into String(format string="Copy Plot to %s\n", initial string=w388, error in=w384, w382) -> (resulting string=w381:string, error out=w379:errorcluster)
          n159 = call "Get Notebook Queue.vi"() -> ("Notebook Queue"=w385:refnum<queue>)  [unwired: 9 in]
          n160 = Format Into String(format string="Plot %s edited:%s", error in=w379, w404, w381) -> (resulting string=w386:string, error out=w378:errorcluster)  [unwired: 1 in]
          n161 = call "XY Graph Get-Set Plot Style.vi"("Error In"=w379, "Plot Index"=w396, "Plot Style in"=w397, "XYGraph in"=w398) -> ("Error Out"=w399:errorcluster)  [unwired: 4 in, 3 out]
          n162 = call "Message Style.vi"() -> ("Message Formatting"=w387:T8)
          n163 = call "Send Message to Notebook.vi"("Notebook Queue"=w385, "Message"=w386, "Error In"=w378, "Text Formatting"=w387) -> ()  [unwired: 15 in, 1 out]
        }
        frame "Save Plot" {
          w416 = T10 3 items=["no dialog", "OK message", "continue or stop message", "OK message + warnings", "continue/stop + warnings"] ("type of dialog (OK msg:1)")
          n164 = call "XY Graph Save Plot.vi"("Error In"=w418, "Plot Index"=0, "XYGraph Ref"=w419) -> ("Error Out"=w409:errorcluster, "File Path"=w411:path)  [unwired: 3 in, 4 out]
          n165 = Format Into String(format string="Plot saved to %s\n", initial string=w413, error in=w409, w411) -> (resulting string=w410:string, error out=w408:errorcluster)
          n166 = call <vilib>:"Simple Error Handler.vi"("type of dialog (OK msg:1)"=w416, "error in (no error)"=w408) -> ("error out"=w417:errorcluster)  [unwired: 3 in, 4 out]
          n167 = call <vilib>:"Clear Errors.vi"("error in (no error)"=w417) -> ("error out"=w415:errorcluster)  [unwired: 5 in, 1 out]
        }
        frame "Load Plot" {
          w437 = T10 3 items=["no dialog", "OK message", "continue or stop message", "OK message + warnings", "continue/stop + warnings"] ("type of dialog (OK msg:1)")
          w427 = 1 ("Max Number of Plot to Load (-1: All)")
          n168 = call "XY Graph Load Plot(s) Event.vi"("Max Number of Plot to Load (-1: All)"=w427, "Error In"=w439, "XYGraph Ref"=w431) -> ("Error Out"=w433:errorcluster, "Message"=w423:string, "File Path(s)"=w424:path[], "# Plots Added"=w435:i32[])  [unwired: 3 in, 2 out]
          n169 = Add Array Elements(numeric array=w435) -> (sum=w434:i32)
          n170 = Equal?(x=w434, y=w427) -> (x = y?=w430:bool)
          n171 = case shown="True" w430 {
            tunnel: w433 -> [w442 w451]
            tunnel: [w442 w448] -> w432
            tunnel: w431 -> [_ w447]
            tunnel: w429 -> [w443 w446]
            tunnel: [w443 w445] -> w428
            tunnel: w426 -> [w441 w455]
            tunnel: [w441 w454] -> w425
            tunnel: w424 -> [_ _]
            tunnel: w423 -> [_ w453]
            tunnel: w422 -> [_ w444]
            frame False {
            }
            frame True {
              # "removes previous plot & updates data"
              n172 = Format Into String(format string="%s\n", initial string=w455, error in=w451, w453) -> (resulting string=w454:string, error out=w452:errorcluster)
              n173 = call "XY Graph Delete Plot.vi"("Error In"=w452, "Plot Index"=0, "XYGraph Ref"=w447) -> ("Error Out"=w449:errorcluster)  [unwired: 5 in, 3 out]
              n174 = call "Plot Editor_Plot to Data & Controls.vi"("Control Refnums"=w444, "XYGraph in"=w447, "error in (no error)"=w449, "Plot Editor Internal Data in"=w446) -> ("error out"=w448:errorcluster, "Plot Editor Internal Data out"=w445:T6)  [unwired: 6 in]
            }
          }
          n175 = call <vilib>:"Simple Error Handler.vi"("type of dialog (OK msg:1)"=w437, "error in (no error)"=w432) -> ("error out"=w438:errorcluster)  [unwired: 3 in, 4 out]
          n176 = call <vilib>:"Clear Errors.vi"("error in (no error)"=w438) -> ("error out"=w436:errorcluster)  [unwired: 5 in, 1 out]
        }
        frame "Remove out-of-bound Values" {
          n177 = call "Plot Editor_Remove out-of-bound Plot Values.vi"("Control Refnums"=w457, "XYGraph in"=w462, "error in (no error)"=w468, "Plot Editor Internal Data"=w459) -> ("error out"=w464:errorcluster, "Message"=w461:string, "Plot Editor Internal Data out"=w458:T6)  [unwired: 5 in]
          n178 = Format Into String(format string="%s\n", initial string=w467, error in=w464, w461) -> (resulting string=w466:string, error out=w463:errorcluster)
        }
        frame "Delete Element", Default {
          n179 = Variant To Data(error in=w473, type=cluster{"CtlRef":refnum<vi>, "Coords":T7} {"CtlRef"=refnum, "Coords"={"Horizontal"=0, "Vertical"=0}} ("output cluster"), Variant=w488) -> (data=w486:cluster{"CtlRef":refnum<vi>, "Coords":T7}, error out=w479:errorcluster)
          n180 = Unbundle(w486) -> ("CtlRef"=w485:refnum<vi>, "Coords"=w484:T7)
          n181 = call "Determine Clicked Array Element Index.vi"("Error In"=w479, "Coords of Click"=w484, "Array Refnum"=w485) -> ("Error Out"=w480:errorcluster, "Clicked Row"=w483:i32)  [unwired: 1 in, 6 out]
          n182 = case shown="0, Default" w483 {
            selector: w483 -> [w500 _]
            tunnel: w482 -> [w509 _]
            tunnel: w481 -> [w508 _]
            tunnel: w480 -> [w502 w511]
            tunnel: w478 -> [w504 w513]
            tunnel: [w503 w513] -> w477
            tunnel: w476 -> [w498 w512]
            tunnel: [w498 w512] -> w475
            tunnel: [w492 w511] -> w474
            tunnel: w472 -> [w496 w510]
            tunnel: w471 -> [w489 _]
            tunnel: w470 -> [w494 _]
            tunnel: [w495 w510] -> w469
            frame 0, Default {
              w505 = 1 ("length")
              n183 = property class="Arr (strict)"(reference=w509, error in=w502) -> (error out=w499:errorcluster, "Value"=w507:dbl[])  [unwired: 1 out]
              n184 = property class="Arr (strict)"(reference=w508, error in=w502) -> (error out=w497:errorcluster, "Value"=w506:dbl[])  [unwired: 1 out]
              n185 = Format Into String(format string="Deleted element %d\n", initial string=w504, error in=w502, w500) -> (resulting string=w503:string)  [unwired: 1 out]
              n186 = Delete From Array(array=w507, length=w505, index=w500) -> (array with subset deleted=w491:dbl[])  [unwired: 1 out]
              n187 = Delete From Array(array=w506, length=w505, index=w500) -> (array with subset deleted=w490:dbl[])  [unwired: 1 out]
              n188 = Merge Errors(w499, w497) -> (w493:errorcluster)
              n189 = call "Plot Editor_Data to Controls & Plot.vi"("Plot Editor Internal Data"=w496, "XYGraph in"=w494, "X Array"=w491, "Y Array"=w490, "error in (no error)"=w493, "Control Refnums"=w489) -> ("Plot Editor Internal Data"=w495:T6, "error out"=w492:errorcluster)  [unwired: 8 in]
            }
            frame -1 {
            }
          }
        }
        frame "Insert Element Before" {
          n190 = Variant To Data(error in=w519, type=cluster{"CtlRef":refnum<vi>, "Coords":T7} {"CtlRef"=refnum, "Coords"={"Horizontal"=0, "Vertical"=0}} ("output cluster"), Variant=w533) -> (data=w531:cluster{"CtlRef":refnum<vi>, "Coords":T7}, error out=w524:errorcluster)
          n191 = Unbundle(w531) -> ("CtlRef"=w530:refnum<vi>, "Coords"=w529:T7)
          n192 = call "Determine Clicked Array Element Index.vi"("Error In"=w524, "Coords of Click"=w529, "Array Refnum"=w530) -> ("Error Out"=w525:errorcluster, "Clicked Row"=w528:i32)  [unwired: 1 in, 6 out]
          n193 = case shown="0, Default" w528 {
            selector: w528 -> [w547 _]
            tunnel: w527 -> [w554 _]
            tunnel: w526 -> [w553 _]
            tunnel: w525 -> [w545 w556]
            tunnel: w523 -> [w549 w558]
            tunnel: [w546 w558] -> w522
            tunnel: w521 -> [w544 w557]
            tunnel: [w544 w557] -> w520
            tunnel: [w538 w556] -> w518
            tunnel: w517 -> [w541 w555]
            tunnel: [w539 w555] -> w516
            tunnel: w515 -> [w540 _]
            tunnel: w514 -> [w534 _]
            frame 0, Default {
              w550 = nan ("new element/subarray")
              n194 = property class="Arr (strict)"(reference=w554, error in=w545) -> (error out=w543:errorcluster, "Value"=w552:dbl[])  [unwired: 1 out]
              n195 = property class="Arr (strict)"(reference=w553, error in=w545) -> (error out=w542:errorcluster, "Value"=w551:dbl[])  [unwired: 1 out]
              n196 = Insert Into Array(array=w552, index=w547, new element=w550) -> (w536:dbl[])
              n197 = Insert Into Array(array=w551, index=w547, new element=w550) -> (w535:dbl[])
              n198 = Format Into String(format string="Element inserted before %d\n", initial string=w549, error in=w545, w547) -> (resulting string=w546:string)  [unwired: 1 out]
              n199 = Merge Errors(w543, w542) -> (w537:errorcluster)
              n200 = call "Plot Editor_Data to Controls & Plot.vi"("Plot Editor Internal Data"=w541, "XYGraph in"=w540, "X Array"=w536, "Y Array"=w535, "error in (no error)"=w537, "Control Refnums"=w534) -> ("Plot Editor Internal Data"=w539:T6, "error out"=w538:errorcluster)  [unwired: 8 in]
            }
            frame -1 {
            }
          }
        }
        frame "Insert Element After" {
          n201 = Variant To Data(error in=w564, type=cluster{"CtlRef":refnum<vi>, "Coords":T7} {"CtlRef"=refnum, "Coords"={"Horizontal"=0, "Vertical"=0}} ("output cluster"), Variant=w578) -> (data=w576:cluster{"CtlRef":refnum<vi>, "Coords":T7}, error out=w571:errorcluster)
          n202 = Unbundle(w576) -> ("CtlRef"=w573:refnum<vi>, "Coords"=w572:T7)
          n203 = call "Determine Clicked Array Element Index.vi"("Error In"=w571, "Coords of Click"=w572, "Array Refnum"=w573) -> ("Error Out"=w570:errorcluster, "Clicked Row"=w569:i32)  [unwired: 1 in, 6 out]
          n204 = case shown="0, Default" w569 {
            selector: w569 -> [w596 _]
            tunnel: w575 -> [w600 _]
            tunnel: w574 -> [w599 _]
            tunnel: w570 -> [w591 w602]
            tunnel: w568 -> [w594 w604]
            tunnel: [w592 w604] -> w567
            tunnel: w566 -> [w582 w603]
            tunnel: [w582 w603] -> w565
            tunnel: [w584 w602] -> w563
            tunnel: w562 -> [w589 w601]
            tunnel: [w583 w601] -> w561
            tunnel: w560 -> [w579 _]
            tunnel: w559 -> [w580 _]
            frame 0, Default {
              w595 = nan ("new element/subarray")
              n205 = property class="Arr (strict)"(reference=w600, error in=w591) -> (error out=w587:errorcluster, "Value"=w598:dbl[])  [unwired: 1 out]
              n206 = property class="Arr (strict)"(reference=w599, error in=w591) -> (error out=w586:errorcluster, "Value"=w597:dbl[])  [unwired: 1 out]
              n207 = Increment(x=w596) -> (x+1=w590:i32)
              n208 = Insert Into Array(array=w598, index=w590, new element=w595) -> (w588:dbl[])
              n209 = Format Into String(format string="Element inserted after %d\n", initial string=w594, error in=w591, w590) -> (resulting string=w592:string)  [unwired: 1 out]
              n210 = Insert Into Array(array=w597, index=w590, new element=w595) -> (w581:dbl[])
              n211 = Merge Errors(w587, w586) -> (w585:errorcluster)
              n212 = call "Plot Editor_Data to Controls & Plot.vi"("Plot Editor Internal Data"=w589, "XYGraph in"=w580, "X Array"=w588, "Y Array"=w581, "error in (no error)"=w585, "Control Refnums"=w579) -> ("Plot Editor Internal Data"=w583:T6, "error out"=w584:errorcluster)  [unwired: 8 in]
            }
            frame -1 {
            }
          }
        }
        frame "Update output string" {
          n213 = call "Variant to String.vi"("Variant"=w612) -> ("String"=w606:string)  [unwired: 8 in]
          n214 = Format Into String(format string="%s\n", initial string=w611, error in=w607, w606) -> (resulting string=w610:string, error out=w608:errorcluster)
        }
        frame "Remove NaN-containing Pairs" {
          n215 = call "Variant to I32.vi"("Variant"=w629) -> ()  [unwired: 8 in, 1 out]
          n216 = Unbundle By Name(w617) -> ("X Array"=w628:dbl[], "Y Array"=w627:dbl[])
          n217 = call "Remove NaN-containing Pairs.vi"("Error In"=w623, "Y Array in"=w627, "X Array in"=w628) -> ("Error Out"=w622:errorcluster, "Y Array out"=w619:dbl[], "# X elts deleted"=w626:i32, "X Array out"=w620:dbl[])  [unwired: 5 in]
          n218 = case shown="1, Default" w626 {
            selector: w626 -> [_ w645]
            tunnel: [w632 w644] -> w624
            tunnel: w625 -> [w632 w642]
            tunnel: w622 -> [w631 w637]
            tunnel: [w631 w641] -> w621
            tunnel: w620 -> [_ w640]
            tunnel: w619 -> [_ w638]
            tunnel: w617 -> [w630 w639]
            tunnel: w616 -> [_ w636]
            tunnel: [w630 w635] -> w615
            tunnel: w614 -> [_ w634]
            frame 0 {
            }
            frame 1, Default {
              n219 = call "Plot Editor_Data to Controls & Plot.vi"("Plot Editor Internal Data"=w639, "XYGraph in"=w634, "X Array"=w640, "Y Array"=w638, "error in (no error)"=w637, "Control Refnums"=w636) -> ("Plot Editor Internal Data"=w635:T6, "error out"=w633:errorcluster)  [unwired: 8 in]
              n220 = Format Into String(format string="%d NaN-containing pair(s)  removed\n", initial string=w642, error in=w633, w645) -> (resulting string=w644:string, error out=w641:errorcluster)
            }
          }
        }
        frame "Fill Array with Ramp" {
          n221 = call-by-ref "?"("error in (no error)"=w656) -> ("error out"=w650:errorcluster, "OK?"=w655:bool, "Ramp"=w654:dbl[])  [unwired: 10 in, 2 out]
          n222 = case shown="True" w655 {
            tunnel: w658 -> [w662 w681]
            tunnel: [w662 w670] -> w657
            tunnel: w654 -> [_ w676]
            tunnel: w653 -> [w661 w680]
            tunnel: [w661 w679] -> w652
            tunnel: w651 -> [w660 w669]
            tunnel: w650 -> [w659 w668]
            tunnel: [w659 w665] -> w649
            tunnel: [w660 w669] -> w648
            tunnel: w647 -> [_ w664]
            tunnel: w646 -> [_ w663]
            frame False {
            }
            frame True {
              n223 = Array Size(array=w676) -> (size(s)=w675:i32)
              n224 = Decrement(x=w675) -> (x-1=w674:i32)
              n225 = Bundle By Name(cluster=w681, "X Array"=w676) -> (w672:T6)
              n226 = Index Array(array=w676, index #2=w674) -> (element #1=w677:dbl, element #2=w673:dbl)  [unwired: 1 in]
              n227 = call "Plot Editor_Store to Controls.vi"("Error In"=w668, "Control Refnums"=w664, "Plot Editor Internal Data in"=w672) -> ("Error Out"=w667:errorcluster, "Plot Editor Internal Data out"=w671:T6)  [unwired: 7 in]
              n228 = call "Plot Editor_Store to Plot.vi"("XYGraph in"=w663, "Error In"=w667, "Plot Editor Internal Data"=w671) -> ("Error Out"=w666:errorcluster, "Plot Editor Internal Data (dup)"=w670:T6)  [unwired: 7 in]
              n229 = Format Into String(format string="X array filled with ram (%#g...%#g [%d])\n", initial string=w680, error in=w666, w677, w673, w675) -> (resulting string=w679:string, error out=w665:errorcluster)
            }
          }
        }
        frame "Quit" {
          n230 = Unbundle By Name(w687) -> ("Original X Array"=w686:dbl[], "Original Y Array"=w685:dbl[], "Original XY Plot Properties"=w684:T2)
          n231 = Bundle By Name(cluster=w687, "X Array"=w686, "Y Array"=w685) -> (w688:T6)
        }
      }
      n232 = Empty Array?(array=w256) -> (empty?=w255:bool)
    }
    "Error" <- w219
  }
  "Plot Style out" <- w30
  "Error Out" <- w35
  n233 = Unregister For Events(event registration refnum=w25) -> ()  [unwired: 1 in, 1 out]
  n234 = Unbundle By Name(w34) -> ("Refnum based call"=w19:bool, "X Array"=w33:dbl[], "Y Array"=w32:dbl[])
  n235 = Release Queue(queue=w40) -> ()  [unwired: 2 in, 3 out]
  n236 = invoke class="VI" method="FP.Close"(reference=w20) -> (reference out=w17:refnum<vi>, error out=w13:errorcluster)  [unwired: 2 in, 1 out]
  n237 = case shown="False" w19 {
    tunnel: w17 -> [w691 w695]
    tunnel: [w691 w694] -> w16
    tunnel: [w690 w693] -> w14
    tunnel: w13 -> [w690 w692]
    frame False {
    }
    frame True {
      n238 = invoke class="VI" method="Abort VI"(reference=w695, error in=w692) -> (reference out=w694:refnum<vi>, error out=w693:errorcluster)  [unwired: 1 in, 1 out]
    }
  }
  n239 = Bundle("X Array"=w33, "Y Array"=w32) -> (→"Plot out":cluster{"X Array":dbl[], "Y Array":dbl[]})  [unwired: 1 in]
  n240 = Close Reference(reference=w16, error in (no error)=w14) -> (error out=w15:errorcluster)
  n241 = call "Clear Error.vi"("Error In"=w15) -> ()  [unwired: 8 in, 1 out]
